vi "HH_ToColorImage.vi"(0 "Data In":u32[](array[numeric]), 1 "Reset":bool, 2 "Image Array In":i32[][][](array[numeric]), 5 "Data Count":i32, 7 "TCSPC Binning":i32[][](array[numeric]), 9 "Pixel Time (Laser Pulses)":i32, 11 "Trace Bins":i32) -> (3 "Image Array Out":i32[][][](array[numeric]), 6 "Total Photon Count":u64[](array[numeric]), 8 "Trigger Times":u64[](array[numeric]), 13 "Total Oveflow Count":u64, 14 "Num Records Total":i64, 15 "Traces":i32[][](array[numeric]))   [LabVIEW 2009]
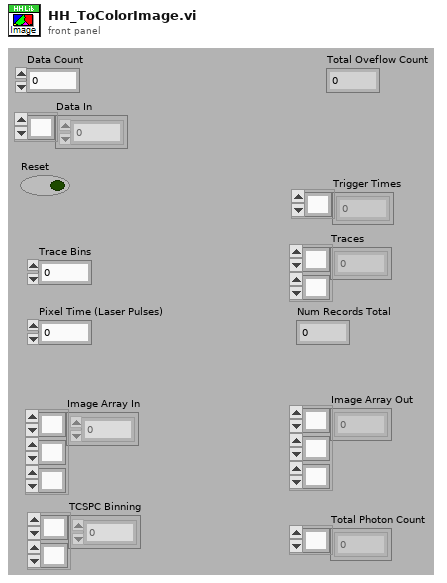
[diagram p1: front panel]
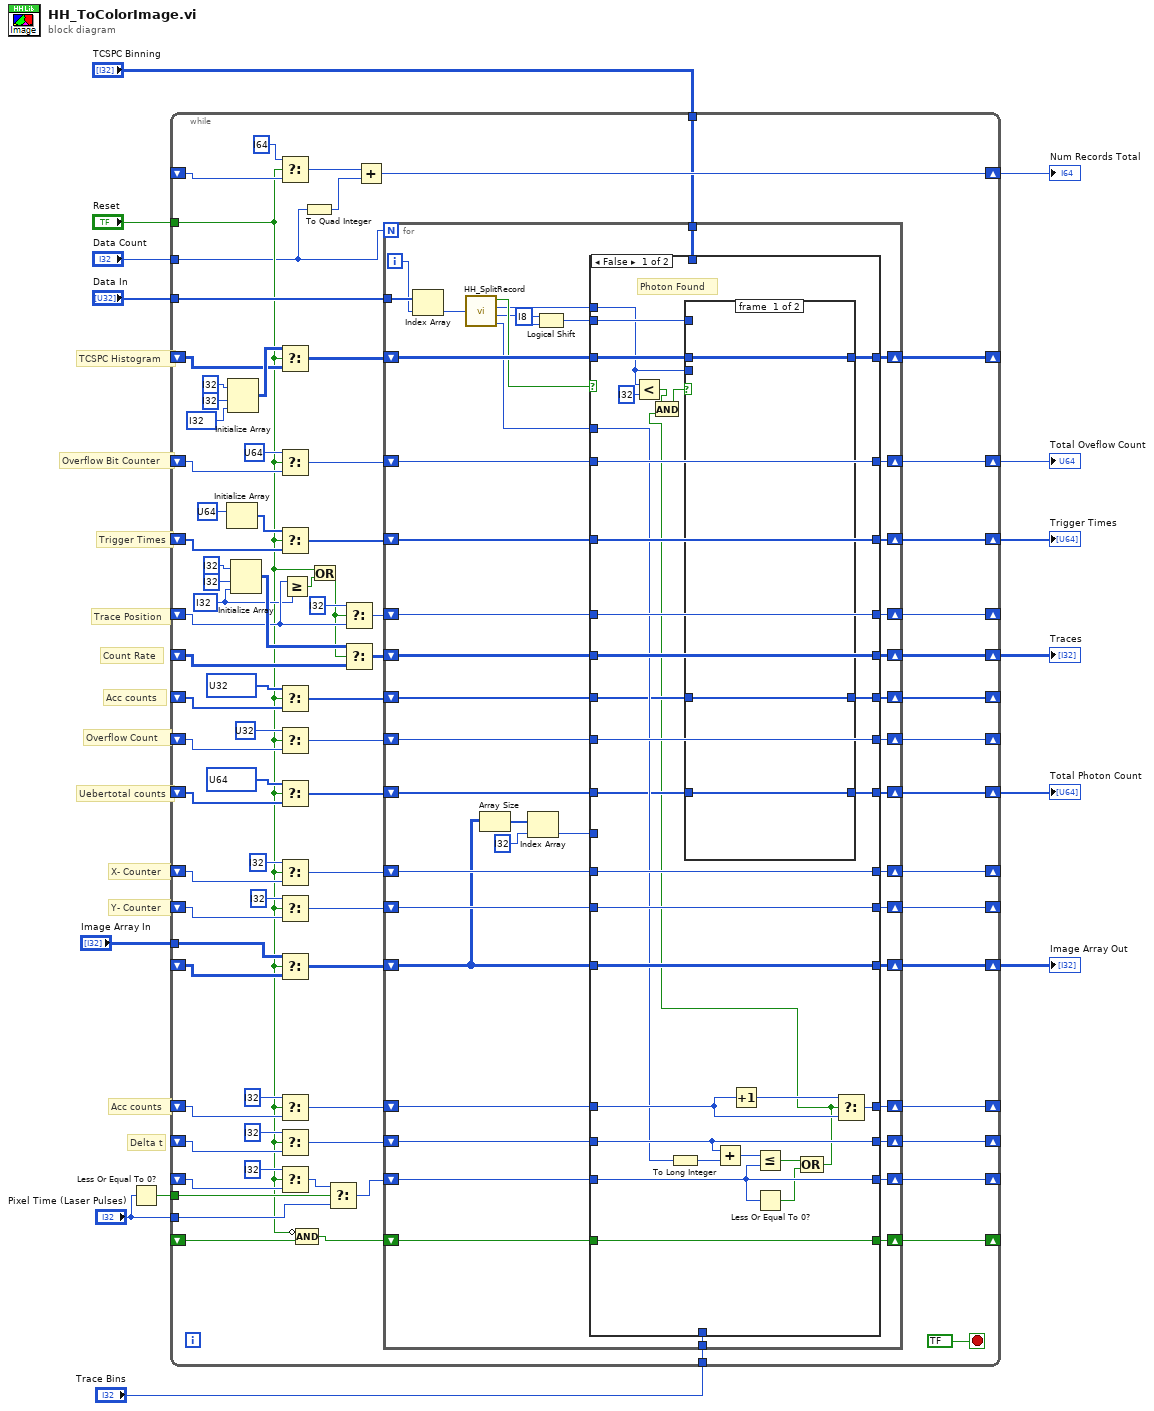
[diagram p0: block diagram]
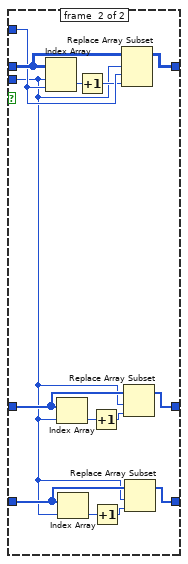
[diagram p2: hidden frame]
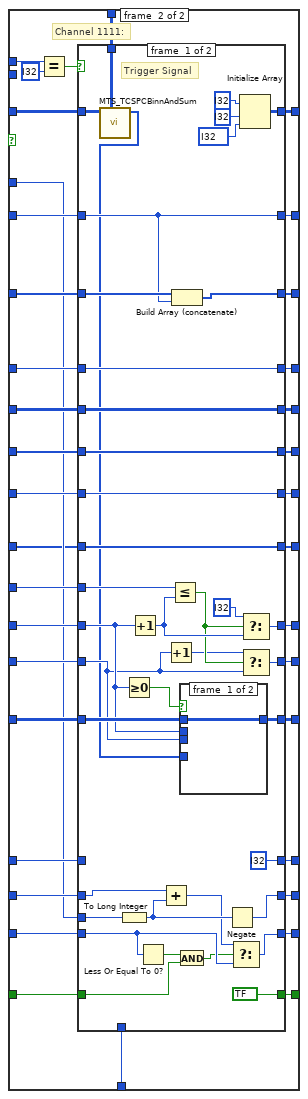
[diagram p3: hidden frame]
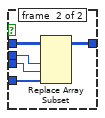
[diagram p4: hidden frame]
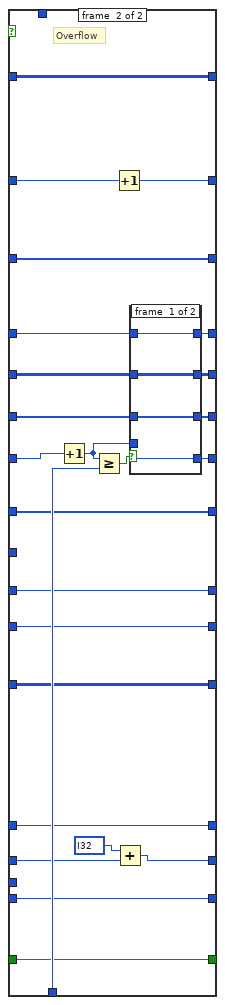
[diagram p5: hidden frame]
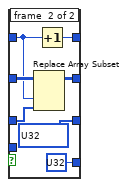
[diagram p6: hidden frame]
diagram:
  # "Uebertotal counts"
  # "Y- Counter"
  # "X- Counter"
  # "Delta t"
  # "Acc counts"
  # "Trace Position"
  # "Overflow Count"
  # "Acc counts"
  # "Count Rate"
  # "Trigger Times"
  # "TCSPC Histogram"
  # "Overflow Bit Counter"
  n1 = Less Or Equal To 0?(x="Pixel Time (Laser Pulses)") -> (x <= 0?=w3:bool)
  n2 = while {
    tunnel: "Data In" -> [w94]
    shift-right: [w95] -> _
    shift-left: _ -> [w90]
    tunnel: "Reset" -> [w18]
    shift-right: [w87] -> w5
    shift-left: _ -> [w86]
    shift-right: [w82] -> w12
    shift-left: _ -> [w81]
    shift-right: [w77] -> w10
    shift-left: _ -> [w76]
    shift-right: [w74] -> _
    shift-left: _ -> [w73]
    shift-right: [w71] -> _
    shift-left: _ -> [w70]
    tunnel: "Trace Bins" -> [w69]
    shift-right: [w66] -> _
    shift-left: _ -> [w64]
    shift-right: [w60] -> w8
    shift-left: _ -> [w59]
    tunnel: "Image Array In" -> [w62]
    shift-right: [w55] -> _
    shift-left: _ -> [w53]
    shift-right: [w54] -> _
    shift-left: _ -> [w52]
    shift-right: [w47] -> _
    shift-left: _ -> [w45]
    shift-right: [w46] -> _
    shift-left: _ -> [w44]
    tunnel: "Data Count" -> [w16]
    shift-right: [w39] -> w6
    shift-left: _ -> [w41]
    shift-right: [w30] -> w4
    shift-left: _ -> [w29]
    shift-right: [w25] -> _
    shift-left: _ -> [w22]
    tunnel: w3 -> [w27]
    tunnel: "Pixel Time (Laser Pulses)" -> [w26]
    shift-right: [w21] -> _
    shift-left: _ -> [w20]
    tunnel: "TCSPC Binning" -> [w17]
    stop <- bool ? stop-if-true
    w36 = i32 ? ("dimension size")
    n3 = Initialize Array(u64 ? ("element")) -> (w84:u64[])  [unwired: 1 out]
    n4 = Initialize Array(i32 ? ("element"), i32 ? ("dimension size"), i32 ? ("dimension size")) -> (w91:i32[][])
    n5 = Initialize Array(i32 ? ("element"), i32 ? ("dimension size"), w36) -> (w79:i32[][])
    n6 = Select(t=i64 ? ("Data Count 2"), s=w18, f=w41) -> (s? t:f=w40:i64)
    n7 = Select(t=w91, s=w18, f=w90) -> (s? t:f=w92:i32[][])
    n8 = Select(t=u64 ?, s=w18, f=w86) -> (s? t:f=w88:u64)
    n9 = Select(t=w84, s=w18, f=w81) -> (s? t:f=w83:u64[])
    n10 = Select(t=u32[] ? ("initialized array"), s=w18, f=w73) -> (s? t:f=w75:u32[])
    n11 = Select(t=u32 ?, s=w18, f=w70) -> (s? t:f=w72:u32)
    n12 = Select(t=u64[] ? ("initialized array"), s=w18, f=w29) -> (s? t:f=w31:u64[])
    n13 = Select(t=i32 ?, s=w18, f=w45) -> (s? t:f=w49:i32)
    n14 = Select(t=i32 ?, s=w18, f=w44) -> (s? t:f=w48:i32)
    n15 = Select(t=w62, s=w18, f=w59) -> (s? t:f=w61:i32[][][])
    n16 = Select(t=i32 ?, s=w18, f=w53) -> (s? t:f=w57:i32)
    n17 = Select(t=i32 ?, s=w18, f=w52) -> (s? t:f=w56:i32)
    n18 = Select(t=i32 ?, s=w18, f=w22) -> (s? t:f=w24:i32)
    n19 = Greater Or Equal?(x=w64, y=w36) -> (x >= y?=w65:bool)
    n20 = Compound Arithmetic op=AND(invert w18, w20) -> (w19:bool)
    n21 = To Quad Integer(1:w16) -> (0:w15:i64)
    n22 = Or(x=w18, y=w65) -> (x .or. y?=w63:bool)
    n23 = Select(t=w24, s=w27, f=w26) -> (s? t:f=w28:i32)
    n24 = Select(t=i32 ?, s=w63, f=w64) -> (s? t:f=w67:i32)
    n25 = Select(t=w79, s=w63, f=w76) -> (s? t:f=w78:i32[][])
    n26 = Add(x=w40, y=w15) -> (x+y=w39:i64)
    n27 = for {
      N: w16 -> [_]
      tunnel: w94 -> [w112]
      shift-right: [w139] -> w95
      shift-left: w92 -> [w140]
      shift-right: [w137] -> w87
      shift-left: w88 -> [w138]
      shift-right: [w135] -> w82
      shift-left: w83 -> [w136]
      shift-right: [w131] -> w77
      shift-left: w78 -> [w132]
      shift-right: [w133] -> w74
      shift-left: w75 -> [w134]
      shift-right: [w129] -> w71
      shift-left: w72 -> [w130]
      tunnel: w69 -> [w128]
      shift-right: [w126] -> w66
      shift-left: w67 -> [w127]
      shift-right: [w125] -> w60
      shift-left: w61 -> [w117]
      shift-right: [w123] -> w55
      shift-left: w57 -> [w124]
      shift-right: [w121] -> w54
      shift-left: w56 -> [w122]
      shift-right: [w118] -> w47
      shift-left: w49 -> [w119]
      shift-right: [w114] -> w46
      shift-left: w48 -> [w120]
      shift-right: [w109] -> w30
      shift-left: w31 -> [w110]
      shift-right: [w108] -> w25
      shift-left: w28 -> [w113]
      shift-right: [w107] -> w21
      shift-left: w19 -> [w106]
      tunnel: w17 -> [w104]
      i -> [w111]
      n28 = Index Array(array=w112, index=w111) -> (element=w103:u32)
      n29 = call "HH_SplitRecord.vi"("Record in"=w103) -> ("Special"=w102:bool, "channel"=w99:i32, "time"=w101:i32, "nsync"=w98:u16)
      n30 = Array Size(array=w117) -> (size(s)=w116:i32[])
      n31 = Index Array(array=w116, index=i32 ?) -> (element=w115:i32)
      n32 = Logical Shift(y=i8 ?, x=w101) -> (x << y=w97:i32)
      n33 = case shown="False" w102 {
        tunnel: w140 -> [w171 w194]
        tunnel: w99 -> [w141 w190]
        tunnel: [w170 w193] -> w139
        tunnel: w97 -> [w142 _]
        tunnel: w138 -> [w169 w225]
        tunnel: [w169 w224] -> w137
        tunnel: w136 -> [w168 w223]
        tunnel: [w168 w222] -> w135
        tunnel: w134 -> [w154 w220]
        tunnel: [w153 w216] -> w133
        tunnel: w132 -> [w167 w219]
        tunnel: [w167 w215] -> w131
        tunnel: w130 -> [w166 w221]
        tunnel: [w166 w217] -> w129
        tunnel: w128 -> [_ w218]
        tunnel: w127 -> [w165 w214]
        tunnel: [w165 w213] -> w126
        tunnel: w117 -> [w164 w211]
        tunnel: [w164 w212] -> w125
        tunnel: w124 -> [w163 w207]
        tunnel: [w162 w208] -> w123
        tunnel: w122 -> [w161 w210]
        tunnel: [w161 w209] -> w121
        tunnel: w120 -> [w160 w206]
        tunnel: w119 -> [w159 w205]
        tunnel: [w159 w204] -> w118
        tunnel: w115 -> [_ w203]
        tunnel: [w160 w202] -> w114
        tunnel: w113 -> [w149 w198]
        tunnel: w98 -> [w156 w201]
        tunnel: w110 -> [w151 w200]
        tunnel: [w150 w199] -> w109
        tunnel: [w149 w197] -> w108
        tunnel: [w146 w196] -> w107
        tunnel: w106 -> [w146 w195]
        tunnel: w104 -> [_ w192]
        frame #0 {
          # "Photon Found"
          n34 = Less?(x=w141, y=i32 ?) -> (x < y?=w145:bool)
          n35 = To Long Integer(number=w156) -> (32bit integer=w155:i32)
          n36 = Add(x=w161, y=w155) -> (x+y=w157:i32)
          n37 = Increment(x=w163) -> (x+1=w158:i32)
          n38 = Less Or Equal?(x=w157, y=w149) -> (x <= y?=w148:bool)
          n39 = Less Or Equal To 0?(x=w149) -> (x <= 0?=w147:bool)
          n40 = Compound Arithmetic op=OR(w148, w147) -> (w143:bool)
          n41 = And(x=w145, y=w143) -> (x .and. y?=w144:bool)
          n42 = case shown="True" w144 {
            tunnel: w171 -> [w174 w188]
            tunnel: [w174 w187] -> w170
            tunnel: w142 -> [_ w186]
            tunnel: w141 -> [_ w175]
            tunnel: w154 -> [w173 w185]
            tunnel: [w173 w184] -> w153
            tunnel: w151 -> [w172 w177]
            tunnel: [w172 w176] -> w150
            frame #0 {
            }
            frame #1 {
              n43 = Index Array(array=w188, index (row)=w175, index (col)=w186) -> (element=w183:i32)
              n44 = Index Array(array=w185, index=w175) -> (element=w181:u32)
              n45 = Index Array(array=w177, index=w175) -> (element=w179:u64)
              n46 = Increment(x=w183) -> (x+1=w182:i32)
              n47 = Increment(x=w181) -> (x+1=w180:u32)
              n48 = Increment(x=w179) -> (x+1=w178:u64)
              n49 = Replace Array Subset(array=w188, new element=w182, index (row)=w175, index (col)=w186) -> (w187:i32[][])
              n50 = Replace Array Subset(array=w185, new element=w180, index=w175) -> (w184:u32[])
              n51 = Replace Array Subset(array=w177, new element=w178, index=w175) -> (w176:u64[])
            }
          }
          n52 = Select(t=w158, s=w143, f=w163) -> (s? t:f=w162:i32)
        }
        frame #1 {
          # "Channel 1111:"
          n53 = Equal?(x=w190, y=i32 ?) -> (x = y?=w189:bool)
          n54 = case shown="True" w189 {
            tunnel: w225 -> [w262 w294]
            tunnel: [w262 w293] -> w224
            tunnel: w223 -> [w264 w295]
            tunnel: [w263 w295] -> w222
            tunnel: w221 -> [w261 w278]
            tunnel: w220 -> [w260 w289]
            tunnel: w219 -> [w259 w287]
            tunnel: w218 -> [_ w292]
            tunnel: [w261 w290] -> w217
            tunnel: [w260 w288] -> w216
            tunnel: [w259 w286] -> w215
            tunnel: w214 -> [w258 w285]
            tunnel: [w258 w284] -> w213
            tunnel: [w256 w283] -> w212
            tunnel: w211 -> [w257 w283]
            tunnel: w210 -> [w242 w276]
            tunnel: [w244 w271] -> w209
            tunnel: [i32 ? ("t") w281] -> w208
            tunnel: w207 -> [_ w281]
            tunnel: w201 -> [w241 _]
            tunnel: w206 -> [w246 w280]
            tunnel: w205 -> [w251 w279]
            tunnel: [w253 w279] -> w204
            tunnel: w203 -> [w252 _]
            tunnel: [w247 w280] -> w202
            tunnel: w200 -> [w243 w275]
            tunnel: [w243 w275] -> w199
            tunnel: w198 -> [w238 w274]
            tunnel: [w237 w274] -> w197
            tunnel: [bool ? w273] -> w196
            tunnel: w195 -> [w233 w273]
            tunnel: w194 -> [w228 w272]
            tunnel: [w229 w272] -> w193
            tunnel: w192 -> [w227 _]
            frame #0 {
              # "Trigger Signal"
              n55 = call "MTS_TCSPCBinnAndSum.vi"("TCSPC Binning"=w227, "TCSPC Histogram"=w228) -> ("Intensity Values"=w226:i32[])  [unwired: 1 in, 8 out]
              n56 = To Long Integer(number=w241) -> (32bit integer=w240:i32)
              n57 = Greater Or Equal To 0?(x=w251) -> (x >= 0?=w254:bool)
              n58 = Increment(x=w251) -> (x+1=w250:i32)
              n59 = Less Or Equal To 0?(x=w238) -> (x <= 0?=w236:bool)
              n60 = Add(x=w242, y=w240) -> (x+y=w239:i32)
              n61 = Increment(x=w246) -> (x+1=w245:i32)
              n62 = Less Or Equal?(x=w252, y=w250) -> (x <= y?=w248:bool)
              n63 = Build Array (concatenate)(w264, w262) -> (w263:u64[])
              n64 = And(x=w236, y=w233) -> (x .and. y?=w235:bool)
              n65 = case shown="True" w254 {
                tunnel: w257 -> [w265 w270]
                tunnel: [w265 w269] -> w256
                tunnel: w246 -> [_ w268]
                tunnel: w251 -> [_ w267]
                tunnel: w226 -> [_ w266]
                frame #0 {
                }
                frame #1 {
                  n66 = Replace Array Subset(array=w270, new element=w266, index (dim 1)=w267, index (dim 2)=w268) -> (w269:i32[][][])  [unwired: 1 in]
                }
              }
              n67 = Negate(x=w240) -> (-x=w244:i32)
              n68 = Select(t=w239, s=w235, f=w238) -> (s? t:f=w237:i32)
              n69 = Initialize Array(i32 ? ("element"), i32 ? ("dimension size"), i32 ? ("dimension size")) -> (w229:i32[][])
              n70 = Select(t=i32 ?, s=w248, f=w250) -> (s? t:f=w253:i32)
              n71 = Select(t=w245, s=w248, f=w246) -> (s? t:f=w247:i32)
            }
            frame #1 {
              # "Overflow"
              n72 = Increment(x=w278) -> (x+1=w277:u32)
              n73 = Greater Or Equal?(x=w277, y=w292) -> (x >= y?=w291:bool)
              n74 = Increment(x=w294) -> (x+1=w293:u64)
              n75 = Add(x=i32 ? ("t"), y=w276) -> (x+y=w271:i32)
              n76 = case shown="True" w291 {
                tunnel: w277 -> [w299 _]
                tunnel: [w299 u32 ?] -> w290
                tunnel: w289 -> [w298 w304]
                tunnel: [w298 u32[] ? ("initialized array")] -> w288
                tunnel: w287 -> [w297 w305]
                tunnel: [w297 w303] -> w286
                tunnel: w285 -> [w296 w301]
                tunnel: [w296 w302] -> w284
                frame #0 {
                }
                frame #1 {
                  n77 = Replace Array Subset(array=w305, new element=w304, index (col)=w301) -> (w303:i32[][])  [unwired: 1 in]
                  n78 = Increment(x=w301) -> (x+1=w302:i32)
                }
              }
            }
          }
        }
      }
    }
  }
  "Trigger Times" <- w12
  "Traces" <- w10
  "Image Array Out" <- w8
  "Num Records Total" <- w6
  "Total Oveflow Count" <- w5
  "Total Photon Count" <- w4
